vi "Enable.vi"(8 "error in (no error)":errorcluster, 11 "PowerSupply in":refnum<class "PowerSupply.lvclass">) -> (0 "error out":errorcluster, 3 "PowerSupply out":refnum<class "PowerSupply.lvclass">)   [LabVIEW 2020, in "PowerSupply.lvclass"]
uses:
  PowerSupply.lvclass
  <vilib>/DigilentWF/DigilentWF.lvlib
panel:
  in  "s":bool
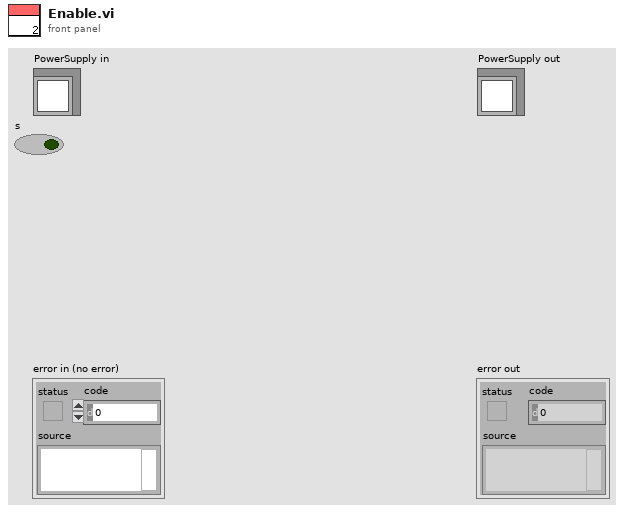
[diagram p1: front panel]
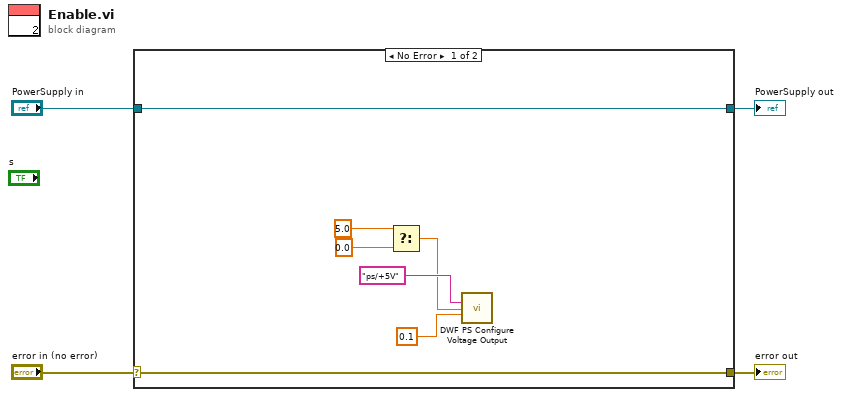
[diagram p0: block diagram]
diagram:
  n1 = case shown="No Error" "error in (no error)" {
    selector: "error in (no error)" -> [w10 w13]
    tunnel: [w10 w13] -> w3
    tunnel: [w11 w12] -> w1
    tunnel: "PowerSupply in" -> [w11 w12]
    frame No Error {
      n2 = Select(t=5.0, f=0.0) -> (s? t:f=w6:dbl)  [unwired: 1 in]
      n3 = call <vilib>:"DWF PS Configure Voltage Output.vi"("Channel"="ps/+5V", "Voltage Level"=w6, "Current Limit"=0.1) -> ()  [unwired: 11 in, 2 out]
    }
    frame Error {
    }
  }
  "error out" <- w3
  "PowerSupply out" <- w1
